vi "CANOpen Recursive Duplicate.vi"(6 "Node ID Name":string, 8 "error in (no error)":errorcluster, 10 "Node Ptr":u64 format="%.0x", 11 "New Node Ptr":u64 format="%.0x") -> (0 "error out":errorcluster)   [LabVIEW 2021, in "CANOpen Addon System Explorer.lvlib"]
uses:
  CANOpen Addon System Explorer.lvlib
  <vilib>/NI VeriStand/Custom Device API/Get Item Property (Variant).vi
  <vilib>/NI VeriStand/Custom Device API/Custom Device API.lvlib
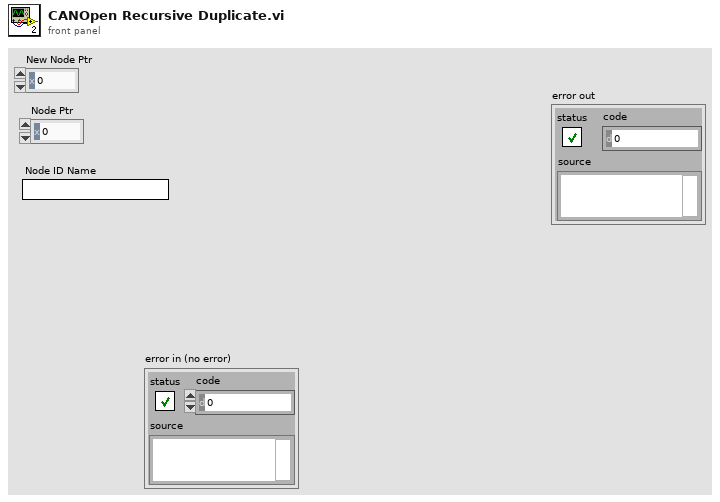
[diagram p1: front panel]
types:
  T1 = typedef "Custom Device API.lvlib/Custom Device Item Info.ctl" = cluster{"Name":string, "Is Channel":bool, "GUID":string, "Is Waveform":bool}
  T2 = typedef "Custom Device API.lvlib/Custom Device Item Ref.ctl" = u64
  T3 = typedef "Custom Device API.lvlib/Custom Device Channel.ctl" = cluster{"Type":T4, "Units":string, "Default Value":dbl, "Faultable":bool, "Scalable":bool}
  T4 = typedef "Custom Device API.lvlib/Custom Device Channel Type.ctl" = enum16{"Input", "Output"}
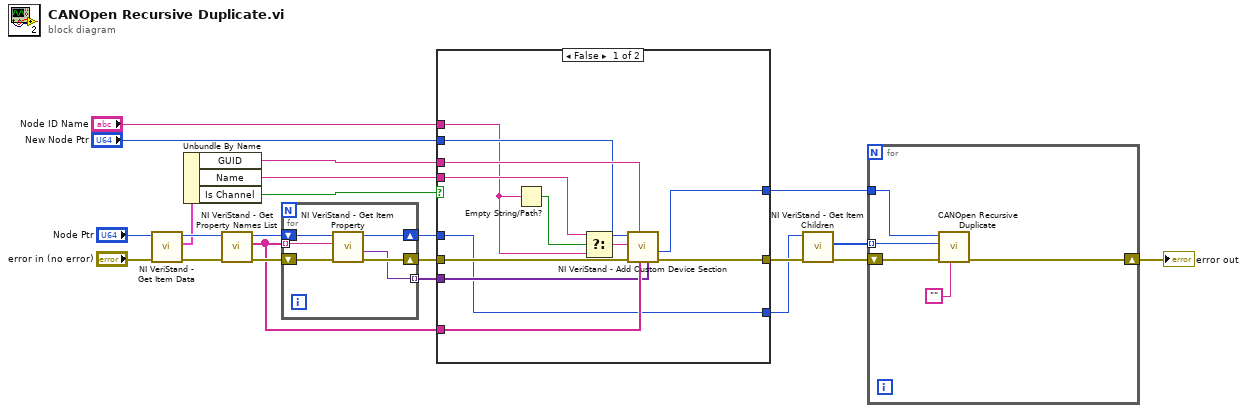
[diagram p0: block diagram]
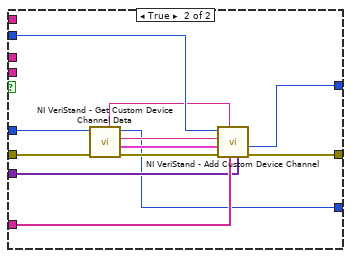
[diagram p2: hidden frame]
diagram:
  n1 = call <vilib>:"NI VeriStand - Get Item Data.vi"("error in (no error)"="error in (no error)", "Item Ref in"="Node Ptr") -> ("error out"=w21:errorcluster, "Item Info"=w17:T1, "Item Ref out"=w20:T2)  [unwired: 6 in, 1 out]
  n2 = Unbundle By Name(w17) -> ("GUID"=w15:string, "Name"=w12:string, "Is Channel"=w11:bool)
  n3 = call <vilib>:"NI VeriStand - Get Property Names List.vi"("error in (no error)"=w21, "Item Ref in"=w20) -> ("error out"=w19:errorcluster, "Property Names"=w14:string[], "Item Ref out"=w18:T2)  [unwired: 7 in]
  n4 = for {
    tunnel: w14 -> [w25] mode=indexing
    shift-right: [w26] -> w16
    shift-left: w19 -> [w28]
    tunnel: [w24] -> w13 mode=indexing
    shift-right: [w23] -> w10
    shift-left: w18 -> [w27]
    n5 = call-poly <vilib>:"NI VeriStand - Get Item Property.vi"("error in (no error)"=w28, "Property Name"=w25, "Item Ref in"=w27) -> ("error out"=w26:errorcluster, "Value"=w24:variant, "Item Ref out"=w23:T2)  [unwired: 5 in, 1 out]
  }
  n6 = case shown="False" w11 {
    tunnel: w16 -> [w40 w50]
    tunnel: w15 -> [w39 _]
    tunnel: "New Node Ptr" -> [w38 w52]
    tunnel: w14 -> [w37 w45]
    tunnel: w13 -> [w36 w44]
    tunnel: w12 -> [w31 _]
    tunnel: [w35 w43] -> w7
    tunnel: [w34 w42] -> w3
    tunnel: w10 -> [w33 w47]
    tunnel: [w33 w41] -> w6
    tunnel: "Node ID Name" -> [w30 _]
    frame False {
      n7 = Empty String/Path?(string/path=w30) -> (empty?=w32:bool)
      n8 = Select(t=w31, s=w32, f=w30) -> (s? t:f=w29:string)
      n9 = call <vilib>:"NI VeriStand - Add Custom Device Section.vi"("Property Values"=w36, "Property names"=w37, "GUID (Default Section)"=w39, "error in (no error)"=w40, "Section Name"=w29, "Parent Ref in"=w38) -> ("error out"=w35:errorcluster, "Section Ptr"=w34:T2)  [unwired: 2 in, 2 out]
    }
    frame True {
      n10 = call <vilib>:"NI VeriStand - Get Custom Device Channel Data.vi"("error in (no error)"=w50, "Channel Ref in"=w47) -> ("error out"=w49:errorcluster, "Channel"=w51:T3, "Channel Name"=w48:string, "Channel Ref out"=w41:T2, "GUID"=w46:string)  [unwired: 4 in, 1 out]
      n11 = call <vilib>:"NI VeriStand - Add Custom Device Channel.vi"("Property Values"=w44, "Property names"=w45, "GUID (Default Channel)"=w46, "error in (no error)"=w49, "Channel"=w51, "Channel Name"=w48, "Parent Ref in"=w52) -> ("error out"=w43:errorcluster, "Channel Ref"=w42:T2)  [unwired: 1 in, 2 out]
    }
  }
  n12 = call <vilib>:"NI VeriStand - Get Item Children.vi"("error in (no error)"=w7, "Item Ref in"=w6) -> ("error out"=w4:errorcluster, "Child Refs"=w5:T2[])  [unwired: 6 in, 2 out]
  n13 = for {
    tunnel: w5 -> [w56] mode=indexing
    shift-right: [w54] -> w2
    shift-left: w4 -> [w57]
    tunnel: w3 -> [w55]
    n14 = call "CANOpen Recursive Duplicate.vi"("Node ID Name"="", "error in (no error)"=w57, "Node Ptr"=w56, "New Node Ptr"=w55) -> ("error out"=w54:errorcluster)  [unwired: 7 in]
  }
  "error out" <- w2
